vi "Configure Analog Gen Ramp.vi"(4 "Rise Fraction (1 %)":dbl=1.0, 5 "Enable Waveform (T: Enable)":bool=TRUE, 6 "High Amplitude (0 Vp)":dbl, 7 "Low Amplitude (0 Vp)":dbl, 8 "error in (no error)":errorcluster, 9 "Frequency (10 Hz)":dbl=10.0, 10 "Channel (0: A)":i32(ring) items=["A", "B"], 11 "VISA resource name":refnum<visa-resource-name>) -> (0 "error out":errorcluster, 3 "VISA resource name out":refnum<visa-resource-name>)   [LabVIEW 2014, in "Stanford Research SR1.lvlib"]
doc: "Configures the attributes of the Analog Generator Ramp waveform."
uses:
  Stanford Research SR1.lvlib
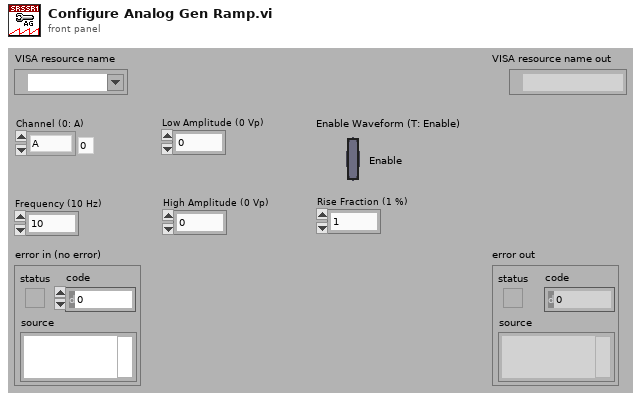
[diagram p1: front panel]
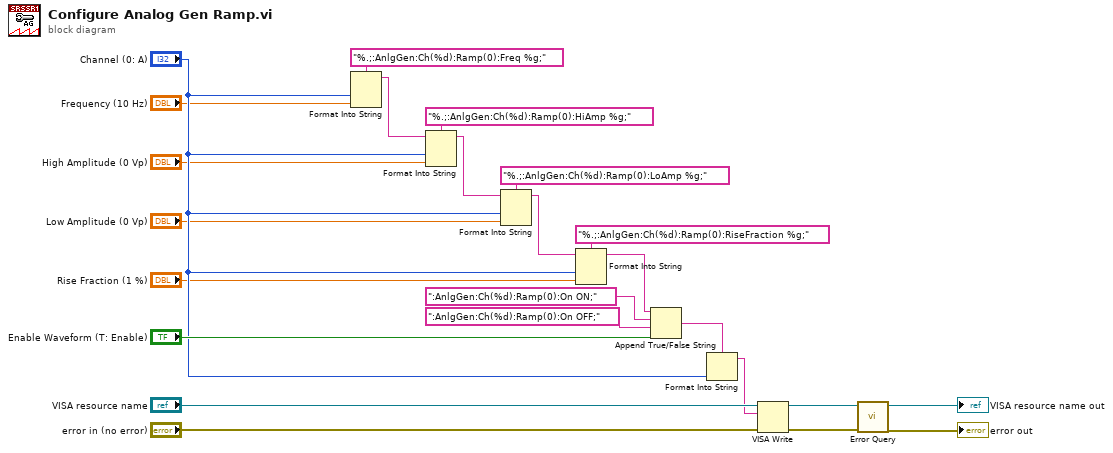
[diagram p0: block diagram]
diagram:
  n1 = Format Into String(format string="%.;:AnlgGen:Ch(%d):Ramp(0):Freq %g;", "Channel (0: A)", "Frequency (10 Hz)") -> (resulting string=w23:string)  [unwired: 2 in, 1 out]
  n2 = Format Into String(format string="%.;:AnlgGen:Ch(%d):Ramp(0):HiAmp %g;", initial string=w23, "Channel (0: A)", "High Amplitude (0 Vp)") -> (resulting string=w21:string)  [unwired: 1 in, 1 out]
  n3 = Format Into String(format string="%.;:AnlgGen:Ch(%d):Ramp(0):LoAmp %g;", initial string=w21, "Channel (0: A)", "Low Amplitude (0 Vp)") -> (resulting string=w19:string)  [unwired: 1 in, 1 out]
  n4 = Format Into String(format string="%.;:AnlgGen:Ch(%d):Ramp(0):RiseFraction %g;", initial string=w19, "Channel (0: A)", "Rise Fraction (1 %)") -> (resulting string=w17:string)  [unwired: 1 in, 1 out]
  n5 = Append True/False String(1:"Enable Waveform (T: Enable)", 2:":AnlgGen:Ch(%d):Ramp(0):On OFF;", 3:":AnlgGen:Ch(%d):Ramp(0):On ON;", 4:w17) -> (0:w7:string)
  n6 = Format Into String(format string=w7, "Channel (0: A)") -> (resulting string=w6:string)  [unwired: 2 in, 1 out]
  n7 = VISA Write(VISA resource name="VISA resource name", write buffer=w6, error in (no error)="error in (no error)") -> (VISA resource name out=w11:refnum<visa-resource-name>, error out=w10:errorcluster)  [unwired: 1 out]
  n8 = call "Error Query.vi"("error in (no error)"=w10, "VISA resource name"=w11) -> ("error out"=→"error out":errorcluster, "VISA resource name out"=→"VISA resource name out":refnum<visa-resource-name>)  [unwired: 6 in, 2 out]
